vi "equalize_trajectory.vi"(0 "TrajectoryTS090820Circular2D in":refnum<class "TrajectoryTS090820Circular2D.lvclass">, 5 "error in (no error)":errorcluster) -> (14 "TrajectoryTS090820Circular2D out":refnum<class "TrajectoryTS090820Circular2D.lvclass">, 15 "x trajectory":dbl[](array[numeric]), 16 "y trajectory":dbl[](array[numeric]), 17 "z trajectory":dbl[](array[numeric]), 18 "intensity":dbl[](array[numeric]), 19 "error out":errorcluster)   [LabVIEW 2010, in "TrajectoryTS090820Circular2D.lvclass"]
uses:
  TrajectoryTS090820Circular2D.lvclass
  <vilib>/Analysis/NI_AALBLAS.lvlib
  <vilib>/Analysis/BLAS.llb/dnrm2 - Vector 2-Norm (DBL).vi
panel:
  out "y trajectory":dbl[](graph)
  out "x trajectory":dbl[](graph)
  out "points AFTER equal-distribution":cluster{dbl, dbl}[](graph)
  out "loop counter":i32
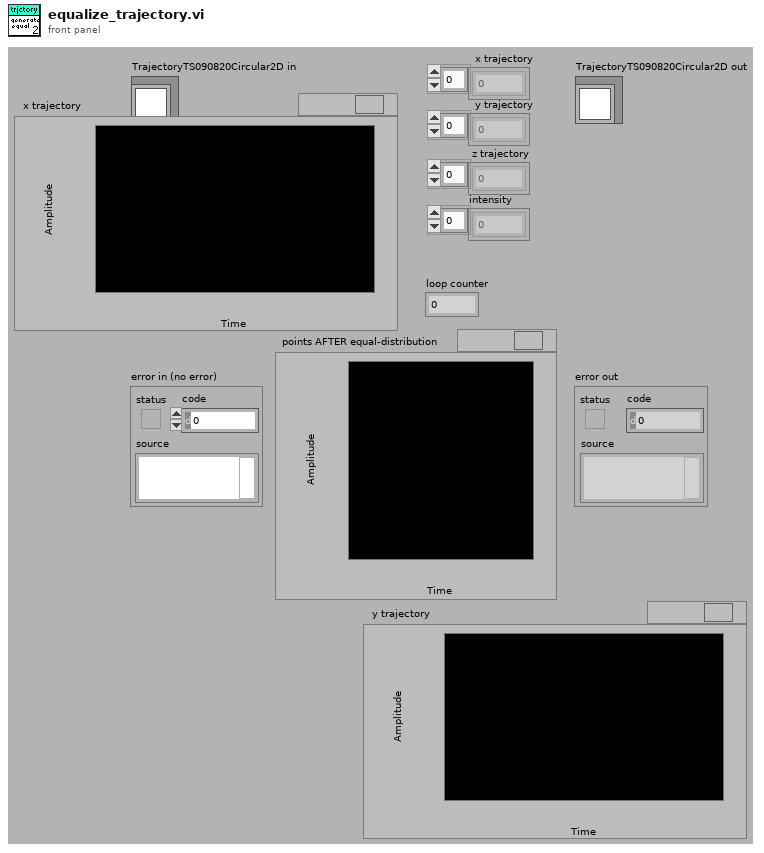
[diagram p1: front panel]
types:
  T1 = cluster{"total number of pixels per cycle":i32, "step":dbl, "x amplitude no units":dbl, "y amplitude no units":dbl, "x frequency":dbl, "y frequency ":dbl, "Phase shift":dbl}
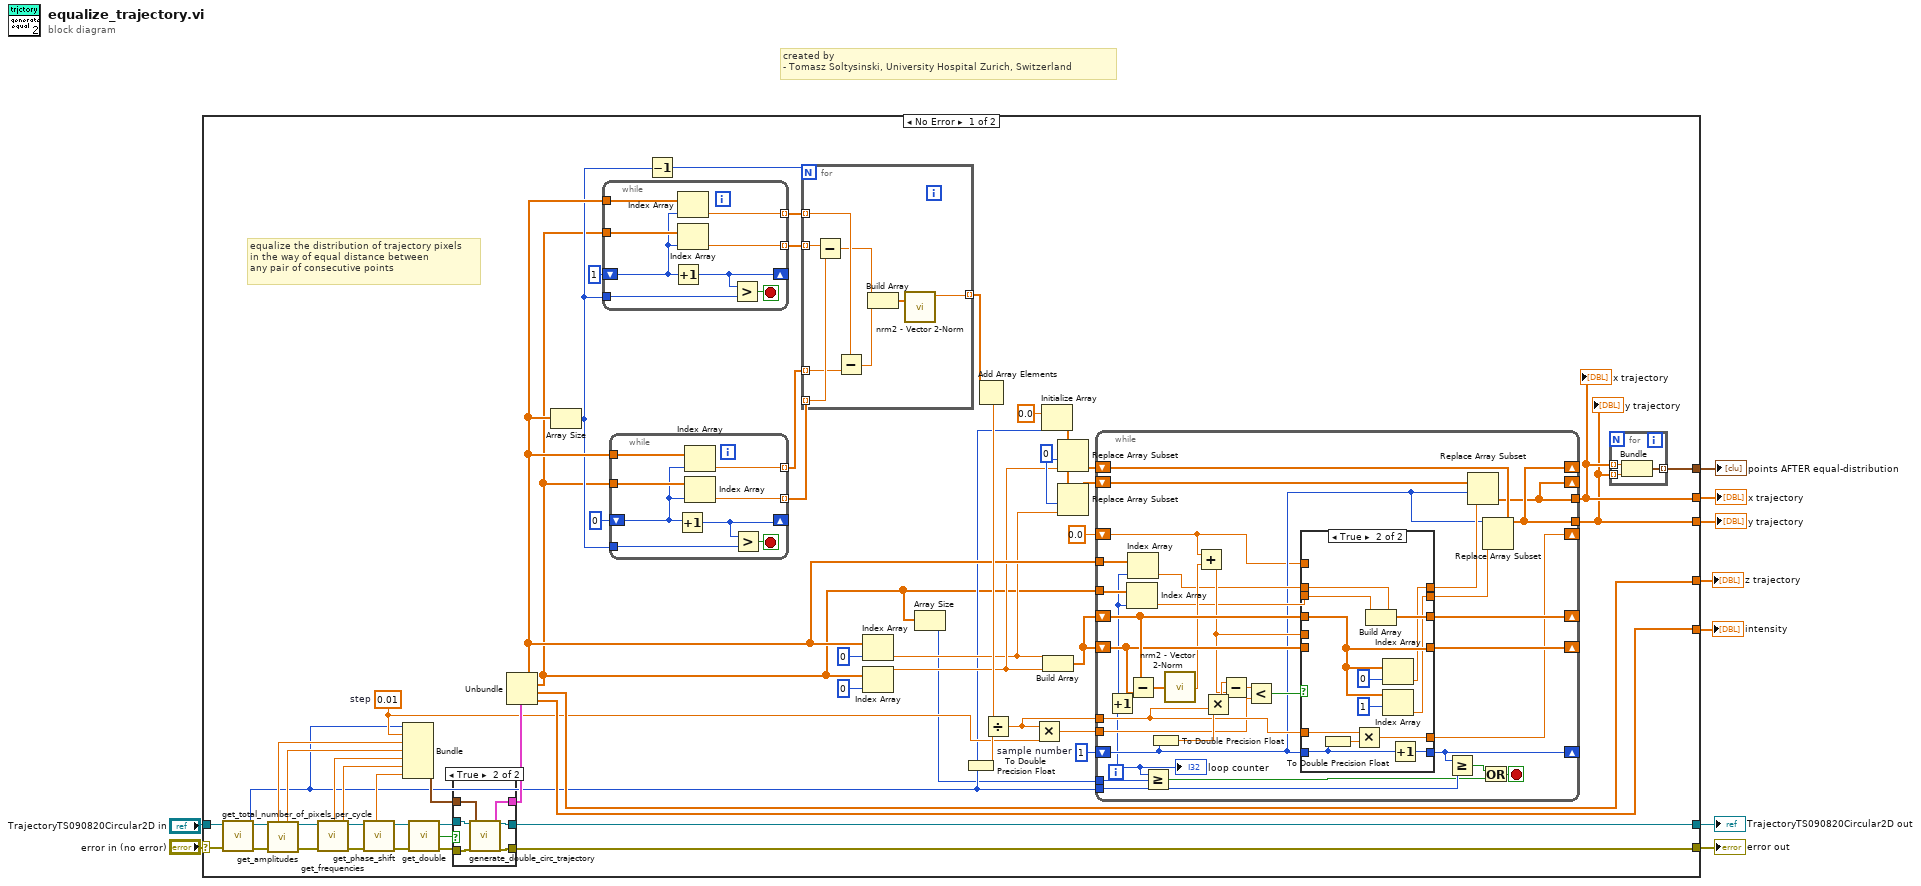
[diagram p0: block diagram]
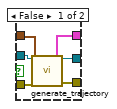
[diagram p2: hidden frame]
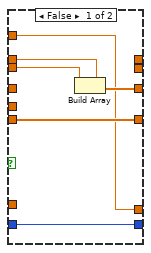
[diagram p3: hidden frame]
diagram:
  # "created by \n- Tomasz Soltysinski, University Hospital Zurich, Switzerland"
  n1 = case shown="No Error" "error in (no error)" {
    selector: "error in (no error)" -> [w64 w160]
    tunnel: [w38 w160] -> w8
    tunnel: [w39 w159] -> w6
    tunnel: "TrajectoryTS090820Circular2D in" -> [w65 w159]
    tunnel: [w25 _] -> w5
    tunnel: [w24 _] -> w4
    tunnel: [w28 _] -> w3
    tunnel: [w27 _] -> w2
    tunnel: [w26 _] -> w1
    frame No Error {
      w34 = 0 ("index")
      w19 = 0.01  # step
      w66 = 1  # sample number
      # "equalize the distribution of trajectory pixels \nin the way of equal distance between \nany pair of consecutive points"
      n2 = call-dynamic "get_total_number_of_pixels_per_cycle.vi"("error in (no error)"=w64, "TrajectoryTS090820Circular2D in"=w65) -> ("error out"=w49:errorcluster, "total number of pixels per cycle"=w17:i32, "TrajectoryTS090820Circular2D out"=w52:refnum<class "TrajectoryTS090820Circular2D.lvclass">)  [unwired: 7 in]
      n3 = call-dynamic "get_amplitudes.vi"("TrajectoryTS090820Circular2D in"=w52, "error in (no error)"=w49) -> ("TrajectoryTS090820Circular2D out"=w51:refnum<class "TrajectoryTS090820Circular2D.lvclass">, "x amplitude no units"=w46:dbl, "y amplitude no units"=w45:dbl, "error out"=w48:errorcluster)  [unwired: 12 in, 2 out]
      n4 = call-dynamic "get_frequencies.vi"("error in (no error)"=w48, "TrajectoryTS090820Circular2D in"=w51) -> ("error out"=w47:errorcluster, "y frequency"=w43:dbl, "x frequency"=w44:dbl, "TrajectoryTS090820Circular2D out"=w50:refnum<class "TrajectoryTS090820Circular2D.lvclass">)  [unwired: 6 in]
      n5 = call-dynamic "get_phase_shift.vi"("error in (no error)"=w47, "TrajectoryTS090820Circular2D in"=w50) -> ("error out"=w14:errorcluster, "Phase shift"=w42:dbl, "TrajectoryTS090820Circular2D out"=w12:refnum<class "TrajectoryTS090820Circular2D.lvclass">)  [unwired: 7 in]
      n6 = Bundle("total number of pixels per cycle"=w17, "step"=w19, "x amplitude no units"=w46, "y amplitude no units"=w45, "x frequency"=w44, "y frequency"=w43, "Phase shift"=w42) -> (w40:T1)  [unwired: 1 in]
      n7 = call-dynamic "get_double.vi"("error in (no error)"=w14, "TrajectoryTS090820Circular2D in"=w12) -> ("error out"=w13:errorcluster, "double"=w10:bool, "TrajectoryTS090820Circular2D out"=w11:refnum<class "TrajectoryTS090820Circular2D.lvclass">)  [unwired: 7 in]
      n8 = case shown="True" w10 {
        tunnel: w11 -> [w72 w78]
        tunnel: w13 -> [w71 w74]
        tunnel: w40 -> [w70 w75]
        tunnel: [w69 w77] -> w39
        tunnel: [w68 w73] -> w38
        tunnel: [w67 w76] -> w33
        frame False {
          n9 = call-dynamic "generate_trajectory.vi"("TrajectoryTS090820Circular2D in"=w72, "trajectory params"=w70, "error in (no error)"=w71) -> ("TrajectoryTS090820Circular2D out"=w69:refnum<class "TrajectoryTS090820Circular2D.lvclass">, "trajectory"=w67:cluster{dbl[], dbl[], dbl[], dbl[]}, "error out"=w68:errorcluster)  [unwired: 14 in]
        }
        frame True {
          n10 = call-dynamic "generate_double_circ_trajectory.vi"("TrajectoryTS090820Circular2D in"=w78, "trajectory params"=w75, "error in (no error)"=w74) -> ("TrajectoryTS090820Circular2D out"=w77:refnum<class "TrajectoryTS090820Circular2D.lvclass">, "trajectory"=w76:cluster{dbl[], dbl[], dbl[], dbl[]}, "error out"=w73:errorcluster)  [unwired: 14 in]
        }
      }
      n11 = Unbundle(w33) -> (w32:dbl[], w16:dbl[], w27:dbl[], w26:dbl[])
      n12 = Array Size(array=w32) -> (size(s)=w30:i32)
      n13 = while {
        shift-right: [w98] -> _
        shift-left: 1 -> [w99]
        tunnel: w16 -> [w100]
        tunnel: [w105] -> w58 mode=indexing
        tunnel: w32 -> [w104]
        tunnel: [w103] -> w31 mode=indexing
        tunnel: w30 -> [w102]
        stop <- w101 stop-if-true
        n14 = Increment(x=w99) -> (x+1=w98:i32)
        n15 = Index Array(array=w104, index=w99) -> (element=w103:dbl)
        n16 = Index Array(array=w100, index=w99) -> (element=w105:dbl)
        n17 = Greater?(x=w98, y=w102) -> (0:w101:bool)
      }
      n18 = while {
        tunnel: w16 -> [w92]
        shift-right: [w90] -> _
        shift-left: 0 -> [w91]
        tunnel: [w97] -> w57 mode=indexing
        tunnel: w32 -> [w96]
        tunnel: [w95] -> w56 mode=indexing
        tunnel: w30 -> [w94]
        stop <- w93 stop-if-true
        n19 = Increment(x=w91) -> (x+1=w90:i32)
        n20 = Index Array(array=w96, index=w91) -> (element=w95:dbl)
        n21 = Index Array(array=w92, index=w91) -> (element=w97:dbl)
        n22 = Greater?(x=w90, y=w94) -> (0:w93:bool)
      }
      n23 = Decrement(x=w30) -> (x-1=w29:i32)
      n24 = for {
        N: w29 -> [_]
        tunnel: w58 -> [w89] mode=indexing
        tunnel: w57 -> [w88] mode=indexing
        tunnel: w56 -> [w87] mode=indexing
        tunnel: w31 -> [w86] mode=indexing
        tunnel: [w82] -> w55 mode=indexing
        n25 = Subtract(x=w89, y=w88) -> (x-y=w84:dbl)
        n26 = Subtract(x=w86, y=w87) -> (x-y=w85:dbl)
        n27 = Build Array(w84, w85) -> (w83:dbl[])
        n28 = call-poly <vilib>:"nrm2 - Vector 2-Norm.vi"("x"=w83) -> ("dnrm2"=w82:dbl)  [unwired: 9 in, 1 out]
      }
      n29 = Index Array(array=w32, index=0) -> (element=w22:dbl)
      n30 = Index Array(array=w16, index=0) -> (element=w23:dbl)
      n31 = Array Size(array=w16) -> (size(s)=w15:i32)
      n32 = To Double Precision Float(number=w17) -> (double precision float=w54:dbl)
      n33 = Add Array Elements(numeric array=w55) -> (sum=w53:dbl)
      n34 = Divide(x=w53, y=w54) -> (x/y=w18:dbl)
      n35 = Multiply(x=w18, y=w19) -> (x*y=w20:dbl)
      n36 = Initialize Array(0.0, w17) -> (w35:dbl[])
      n37 = Build Array(w22, w23) -> (w41:dbl[])
      n38 = Replace Array Subset(array=w35, new element=w23, index=w34) -> (w37:dbl[])
      n39 = Replace Array Subset(array=w35, new element=w22, index=w34) -> (w36:dbl[])
      n40 = while {
        tunnel: w17 -> [w139]
        shift-right: [w132] -> _
        shift-left: w66 -> [w113]
        tunnel: w20 -> [w118]
        shift-right: [w138] -> _
        shift-left: w41 -> [w136]
        shift-right: [w137] -> _
        shift-left: w41 -> [w135]
        tunnel: [w126] -> w25
        tunnel: [w127] -> w24
        shift-right: [w127] -> _
        shift-left: w37 -> [w129]
        shift-right: [w126] -> _
        shift-left: w36 -> [w128]
        tunnel: w32 -> [w117]
        tunnel: w16 -> [w115]
        shift-right: [w125] -> _
        shift-left: 0.0 -> [w111]
        tunnel: w18 -> [w123]
        tunnel: w15 -> [w110]
        i -> [w109]
        stop <- w106 stop-if-true
        n41 = Increment(x=w109) -> (x+1=w112:i32)
        n42 = Index Array(array=w115, index=w112) -> (element=w114:dbl)
        n43 = Index Array(array=w117, index=w112) -> (element=w116:dbl)
        n44 = Subtract(x=w136, y=w135) -> (x-y=w134:dbl[])
        n45 = Greater Or Equal?(x=w109, y=w110) -> (x >= y?=w107:bool)
        n46 = To Double Precision Float(number=w113) -> (double precision float=w124:dbl)
        n47 = call-poly <vilib>:"nrm2 - Vector 2-Norm.vi"("x"=w134) -> ("dnrm2"=w122:dbl)  [unwired: 9 in, 1 out]
        n48 = Add(x=w111, y=w122) -> (x+y=w120:dbl)
        n49 = Multiply(x=w123, y=w124) -> (x*y=w121:dbl)
        n50 = Subtract(x=w121, y=w120) -> (x-y=w119:dbl)
        n51 = Less?(x=w119, y=w118) -> (x < y?=w133:bool)
        n52 = case shown="True" w133 {
          tunnel: w113 -> [w145 w156]
          tunnel: [w145 w158] -> w132
          tunnel: [w143 w157] -> w138
          tunnel: w136 -> [_ w150]
          tunnel: w135 -> [w144 _]
          tunnel: [w144 w150] -> w137
          tunnel: w116 -> [w142 w149]
          tunnel: w114 -> [w141 w147]
          tunnel: [_ w148] -> w131
          tunnel: [_ w146] -> w130
          tunnel: w123 -> [_ w154]
          tunnel: [w140 w153] -> w125
          tunnel: w120 -> [_ _]
          tunnel: w111 -> [w140 _]
          frame False {
            n53 = Build Array(w142, w141) -> (w143:dbl[])
          }
          frame True {
            n54 = To Double Precision Float(number=w156) -> (double precision float=w155:dbl)
            n55 = Multiply(x=w154, y=w155) -> (x*y=w153:dbl)
            n56 = Build Array(w149, w147) -> (w157:dbl[])
            n57 = Index Array(array=w150, index=0) -> (element=w148:dbl)
            n58 = Index Array(array=w150, index=1) -> (element=w146:dbl)
            n59 = Increment(x=w156) -> (x+1=w158:i32)
          }
        }
        n60 = Greater Or Equal?(x=w132, y=w139) -> (x >= y?=w108:bool)
        n61 = Replace Array Subset(array=w128, new element=w131, index=w113) -> (w126:dbl[])
        n62 = Or(x=w108, y=w107) -> (x .or. y?=w106:bool)
        n63 = Replace Array Subset(array=w129, new element=w130, index=w113) -> (w127:dbl[])
        "loop counter" <- w109
      }
      "x trajectory" <- w25
      "y trajectory" <- w24
      n64 = for {
        tunnel: [w81] -> w28 mode=indexing
        tunnel: w25 -> [w80] mode=indexing
        tunnel: w24 -> [w79] mode=indexing
        n65 = Bundle(w80, w79) -> (w81:cluster{dbl, dbl})  [unwired: 1 in]
      }
    }
    frame Error {
    }
  }
  "error out" <- w8
  "TrajectoryTS090820Circular2D out" <- w6
  "x trajectory" <- w5
  "y trajectory" <- w4
  "points AFTER equal-distribution" <- w3
  "z trajectory" <- w2
  "intensity" <- w1
